vi "Utility Format Pressure Compensation.vi"(8 "error in (no error)":errorcluster, 11 "Pressure Compensation (PSI)":i32) -> (0 "error out":errorcluster, 3 "Formatted Compensation":string)   [LabVIEW 2020, in "ChromTech Series III Pump.lvlib"]
doc: "Formats the command to set the User Compensation, given a desired compensation number. This number must be between 85.0 and 115.0, or the function will default to a compensation value of 100.0."
uses:
  <instrlib>/RxnRover/ChromtechSeriesIIIDriver/ChromTech Series III Pump.lvlib
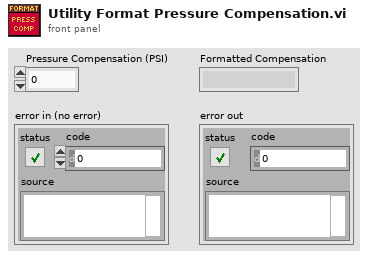
[diagram p1: front panel]
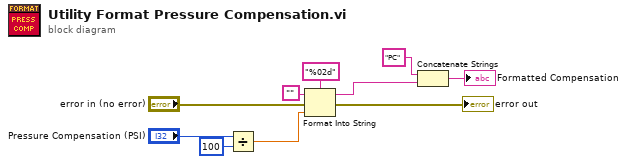
[diagram p0: block diagram]
diagram:
  n1 = Divide(x="Pressure Compensation (PSI)", y=100) -> (x/y=w2:dbl)
  n2 = Format Into String(format string="%02d", initial string="", error in="error in (no error)", w2) -> (resulting string=w6:string, error out=→"error out":errorcluster)
  n3 = Concatenate Strings("PC", w6) -> (→"Formatted Compensation":string)
